vi "行进距离子VI1.vi"(0 "脉冲输入端":i32) -> (1 "行进脉冲总数高位":string, 2 "行进脉冲总数中位":string, 3 "行进脉冲总数低位":string)   [LabVIEW 2014]
panel:
  # "Max=16777214"
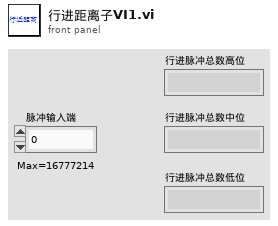
[diagram p1: front panel]
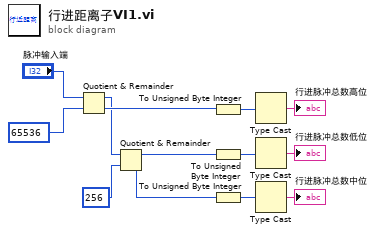
[diagram p0: block diagram]
diagram:
  n1 = Quotient & Remainder(x="脉冲输入端", y=65536) -> (x-y*floor(x/y)=w3:i32, floor(x/y)=w4:i32)
  n2 = Quotient & Remainder(x=w3, y=256) -> (x-y*floor(x/y)=w2:i32, floor(x/y)=w1:i32)
  n3 = To Unsigned Byte Integer(number=w4) -> (unsigned 8bit integer=w11:u8)
  n4 = To Unsigned Byte Integer(number=w2) -> (unsigned 8bit integer=w9:u8)
  n5 = To Unsigned Byte Integer(number=w1) -> (unsigned 8bit integer=w6:u8)
  n6 = Type Cast(x=w11) -> (*(type *) &x=→"行进脉冲总数高位":string)  [unwired: 1 in]
  n7 = Type Cast(x=w9) -> (*(type *) &x=→"行进脉冲总数低位":string)  [unwired: 1 in]
  n8 = Type Cast(x=w6) -> (*(type *) &x=→"行进脉冲总数中位":string)  [unwired: 1 in]
